vi "Launch ECAT Reconfig.vi"(8 "error in (no error)":errorcluster, 11 "ECAT Reconfig VI Ref in":refnum<vi>) -> (0 "error out":errorcluster, 3 "ECAT Reconfig VI Ref out":refnum<vi>)   [LabVIEW 2020, in "SEECD Engine.lvlib"]
uses:
  SEECD Engine.lvlib
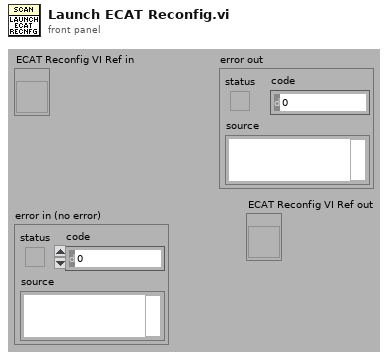
[diagram p1: front panel]
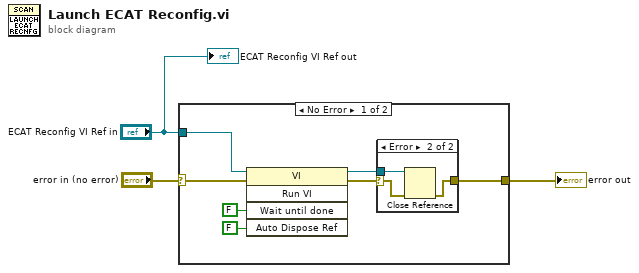
[diagram p0: block diagram]
diagram:
  n1 = case shown="No Error" "error in (no error)" {
    selector: "error in (no error)" -> [w4 w15]
    tunnel: "ECAT Reconfig VI Ref in" -> [w5 _]
    tunnel: [w10 w15] -> w3
    frame No Error {
      n2 = invoke class="VI" method="Run VI"(reference=w5, error in=w4, "Wait until done"=FALSE ("Wait Until Done"), "Auto Dispose Ref"=FALSE ("Auto Dispose Reference")) -> (reference out=w6:refnum<vi>, error out=w7:errorcluster)  [unwired: 1 in, 3 out]
      n3 = case shown="Error" w7 {
        selector: w7 -> [w11 w13]
        tunnel: w6 -> [_ w14]
        tunnel: [w11 w12] -> w10
        frame No Error {
        }
        frame Error {
          n4 = Close Reference(reference=w14, error in (no error)=w13) -> (error out=w12:errorcluster)
        }
      }
    }
    frame Error {
    }
  }
  "error out" <- w3
  "ECAT Reconfig VI Ref out" <- "ECAT Reconfig VI Ref in"
